vi "write write directory.vi"(8 "error in (no error)":errorcluster, 10 "Write Directory":path, 11 "Shared Memory Configuration in":refnum<class "Shared Memory Configuration.lvclass">) -> (0 "error out":errorcluster, 3 "Shared Memory Configuration out":refnum<class "Shared Memory Configuration.lvclass">)   [LabVIEW 2013, in "Shared Memory Configuration.lvclass"]
doc: "Copyright 2016 National Instruments Corporation\n\nLicensed under the Apache License, Version 2.0 (the \"License\"); you may not use this file except in compliance with the License. You may obtain a copy of the License at http://www.apache.org/licenses/LICENSE-2.0\nUnless required by applicable law or agreed to in writing, software distributed under the License is distributed on an \"AS IS\" BASIS, WITHOUT WARRANTIES OR CONDITIONS OF ANY KIND, either express or implied. See the License for the specific language governing permissions and limitations under the License."
uses:
  Shared Memory Configuration.lvclass
  Shared Memory Configuration.lvclass/Shared Memory Configuration.ctl
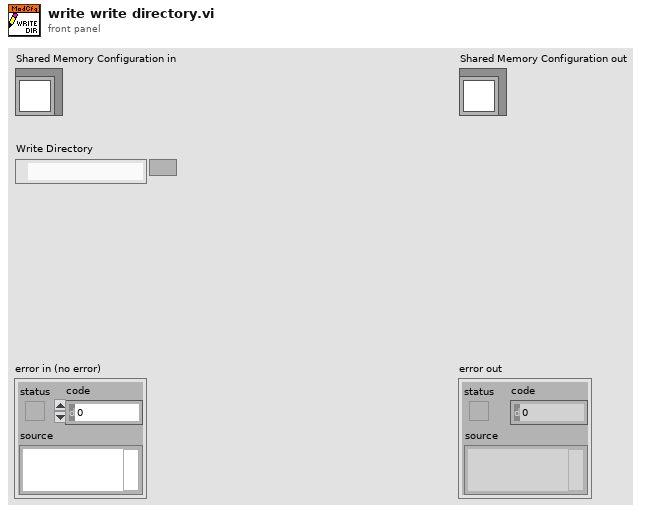
[diagram p1: front panel]
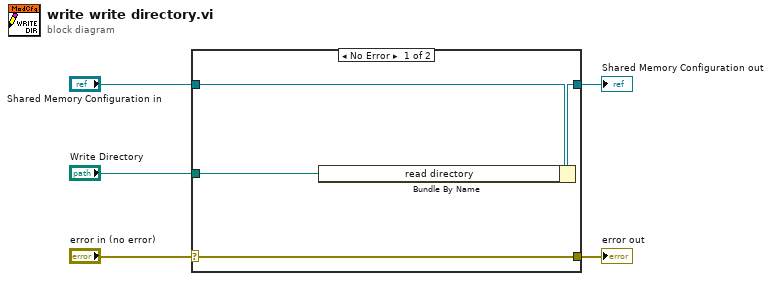
[diagram p0: block diagram]
diagram:
  n1 = case shown="No Error" "error in (no error)" {
    selector: "error in (no error)" -> [w9 w10]
    tunnel: [w9 w10] -> w4
    tunnel: [w7 w11] -> w2
    tunnel: "Shared Memory Configuration in" -> [w8 w11]
    tunnel: "Write Directory" -> [w6 _]
    frame No Error {
      n2 = Bundle By Name(cluster=w8, "read directory"=w6) -> (w7:refnum<class "Shared Memory Configuration.lvclass">)
    }
    frame Error {
    }
  }
  "error out" <- w4
  "Shared Memory Configuration out" <- w2
